vi "DSF.Engine.Get Hardware Info.vi"() -> (3 "Hardware Info":T1 {"CPU"."caches"."cache entry size" format="%d bytes"; "CPU"."caches"."total cache size" format="%d bytes"})   [LabVIEW 2016, in "DSF.Engine.lvlib"]
uses:
  DSF.Engine.lvlib
  Classes/Framework/DSF.Engine.Runtime.Framework.Hardware.ctl
  Classes/Framework/DSF.Engine.Typedefs.CPU Info.ctl
  Classes/Framework/DSF.Engine.Runtime.Framework.lvclass
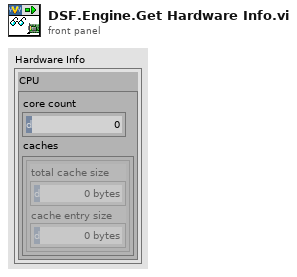
[diagram p1: front panel]
types:
  T1 = typedef "DSF.Engine.lvlib/DSF.Engine.Runtime.Framework.lvclass/DSF.Engine.Runtime.Framework.Hardware.ctl" = cluster{"CPU":T2}
  T2 = typedef "DSF.Engine.lvlib/DSF.Engine.Typedefs.CPU Info.ctl" = cluster{"core count":i32, "caches":cluster{"total cache size":i32, "cache entry size":i32}[]}
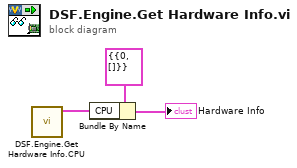
[diagram p0: block diagram]
diagram:
  n1 = call "DSF.Engine.Get Hardware Info.CPU.vi"() -> ("CPU Info"=w1:T2)  [unwired: 11 in]
  n2 = Bundle By Name(cluster=T1 {"CPU"={"core count"=0, "caches"=[]}} ("Hardware Info"), "CPU"=w1) -> (→"Hardware Info":T1)
